vi "运维调试界面.vi"() -> ()   [LabVIEW 2016, in "质控单元V1.lvlib"]
uses:
  <vilib>/Utility/miscctls.llb/LVPointTypeDef.ctl
panel:
  in  "周期设置":bool
  in  "集成干预测试":bool
  in  "平行样测试":bool
  in  "水样测试":bool
  in  "数值":u8
  in  "向前寻道按钮":bool
  in  "向后寻道按钮":bool
  out "质控状态 4":T1
  out "质控状态 3":T1
  out "质控状态 2":T1
  out "质控状态":T1
  out "权限等级":string
  in  "布尔":bool
  out "模块版本号":string
  in  "停止":bool
  in  "参数设置":bool
  in  "连接设置":bool
  in  "调试界面":bool
  in  "加标回收":bool
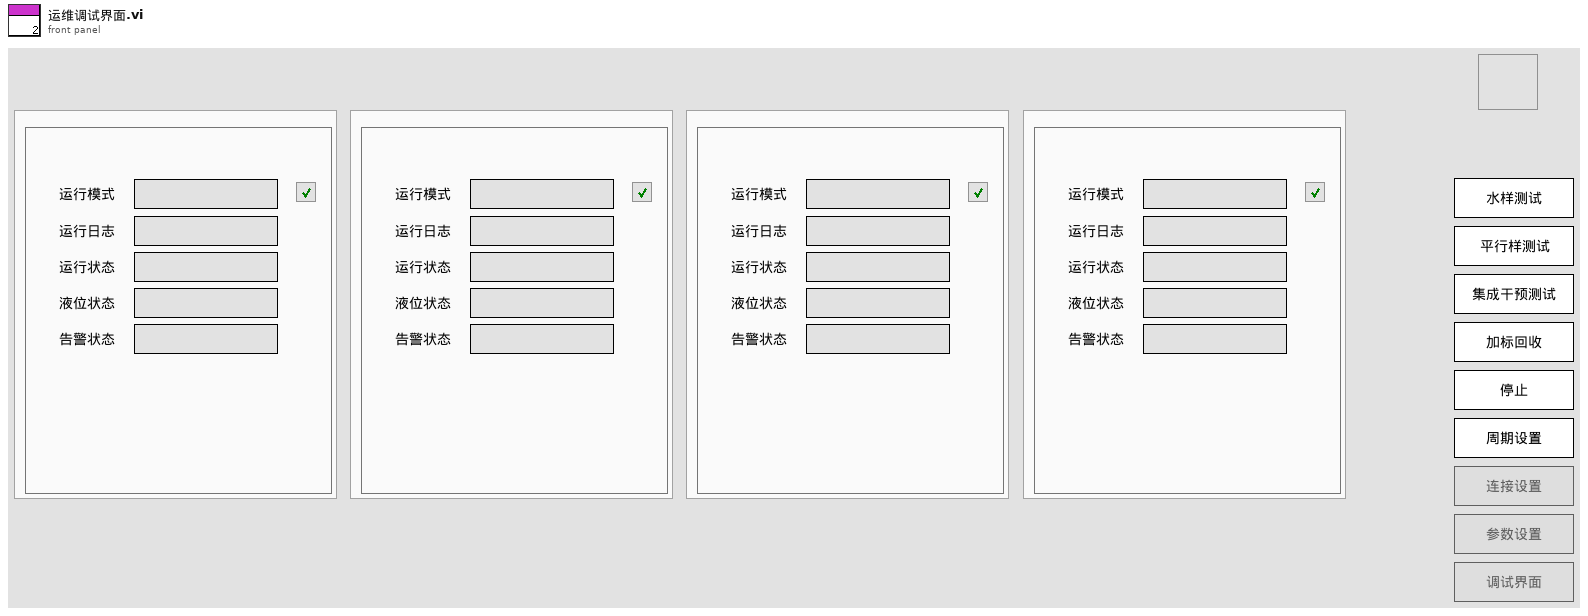
[diagram p1: front panel]
types:
  T1 = typedef "质控单元V1.lvlib/质控状态.ctl" = cluster{"模块名称":string, "通讯状态":bool, "运行模式":string, "运行日志":string, "运行状态":string, "液位状态":string, "告警状态":string}
  T2 = typedef "质控单元V1.lvlib/数据流类型.ctl" = cluster{"cmd":enum16{"start", "stop"}, "data":variant}
  T3 = typedef "LVPointTypeDef.ctl" = cluster{"Horizontal":i16, "Vertical":i16}
  T4 = typedef "质控单元V1.lvlib/质控仪器状态显示.ctl" = cluster{"运行模式":string, "运行状态":string, "液位状态":string, "告警状态":string, "加标体积":string}
  T5 = cluster{"氨氮":bool, "总磷":bool, "总氮":bool, "CODMn":bool, "CODCr":bool, "氨氮总磷":bool, "总磷总氮":bool}
  T6 = typedef "质控单元V1.lvlib/质控slave id.ctl" = enum16{"null", "氨氮", "总磷", "CODMn", "CODCr", "总氮"}
  T7 = typedef "质控单元V1.lvlib/测试流程.ctl" = enum16{"加标回收（启动采配水）", "加标回收（不启动采配水）", "水样测试（启动采配水）", "水样测试（不启动采配水）", "平行样测试（启动采配水）", "平行样测试（不启动采配水）", "集成干预测试"}
  T8 = cluster{"启用参数选择":cluster{"氨氮启用":bool, "总磷启用":bool, "总氮启用":bool, "CODMn启用":bool, "CODCr启用":bool}, "流程":T7}
  T9 = cluster{"氨氮启用":bool, "总磷启用":bool, "总氮启用":bool, "CODMn启用":bool, "CODCr启用":bool}
  T10 = enum8{"Enabled", "Disabled", "Disabled and Grayed Out"}
  T11 = cluster{"Major":u16, "Minor":u16, "Fix":u16, "Build":u16}
  T12 = cluster{"氨氮":bool, "总磷":bool, "总氮":bool, "CODMn":bool, "CODCr":bool}
  T13 = cluster{"氨氮":bool, "总磷":bool, "总氮":bool, "CODMn":bool, "CODCr":bool, bool}
  T14 = typedef "ZKTimingControl.lvlib/TimingControl.lvclass/国标控制命令.ctl" = enum16{"加标回收（启动采配水）", "加标回收（不启动采配水）", "水样测试（启动采配水）", "水样测试（不启动采配水）", "平行样测试（启动采配水）", "平行样测试（不启动采配水）", "集成干预测试"}
  T15 = typedef "ZKTimingControl.lvlib/TimingControl.lvclass/测量参数.ctl" = cluster{"氨氮":bool, "总磷":bool, "总氮":bool, "CODMn":bool, "CODCr":bool, "氟化物":bool}
  T16 = enum32{"Bad", "Idle", "Run top level", "Running"}
  T17 = cluster{"启动参数":cluster{"氨氮启用":bool, "总磷启用":bool, "总氮启用":bool, "CODMn启用":bool, "CODCr启用":bool}, "流程参数":T7}
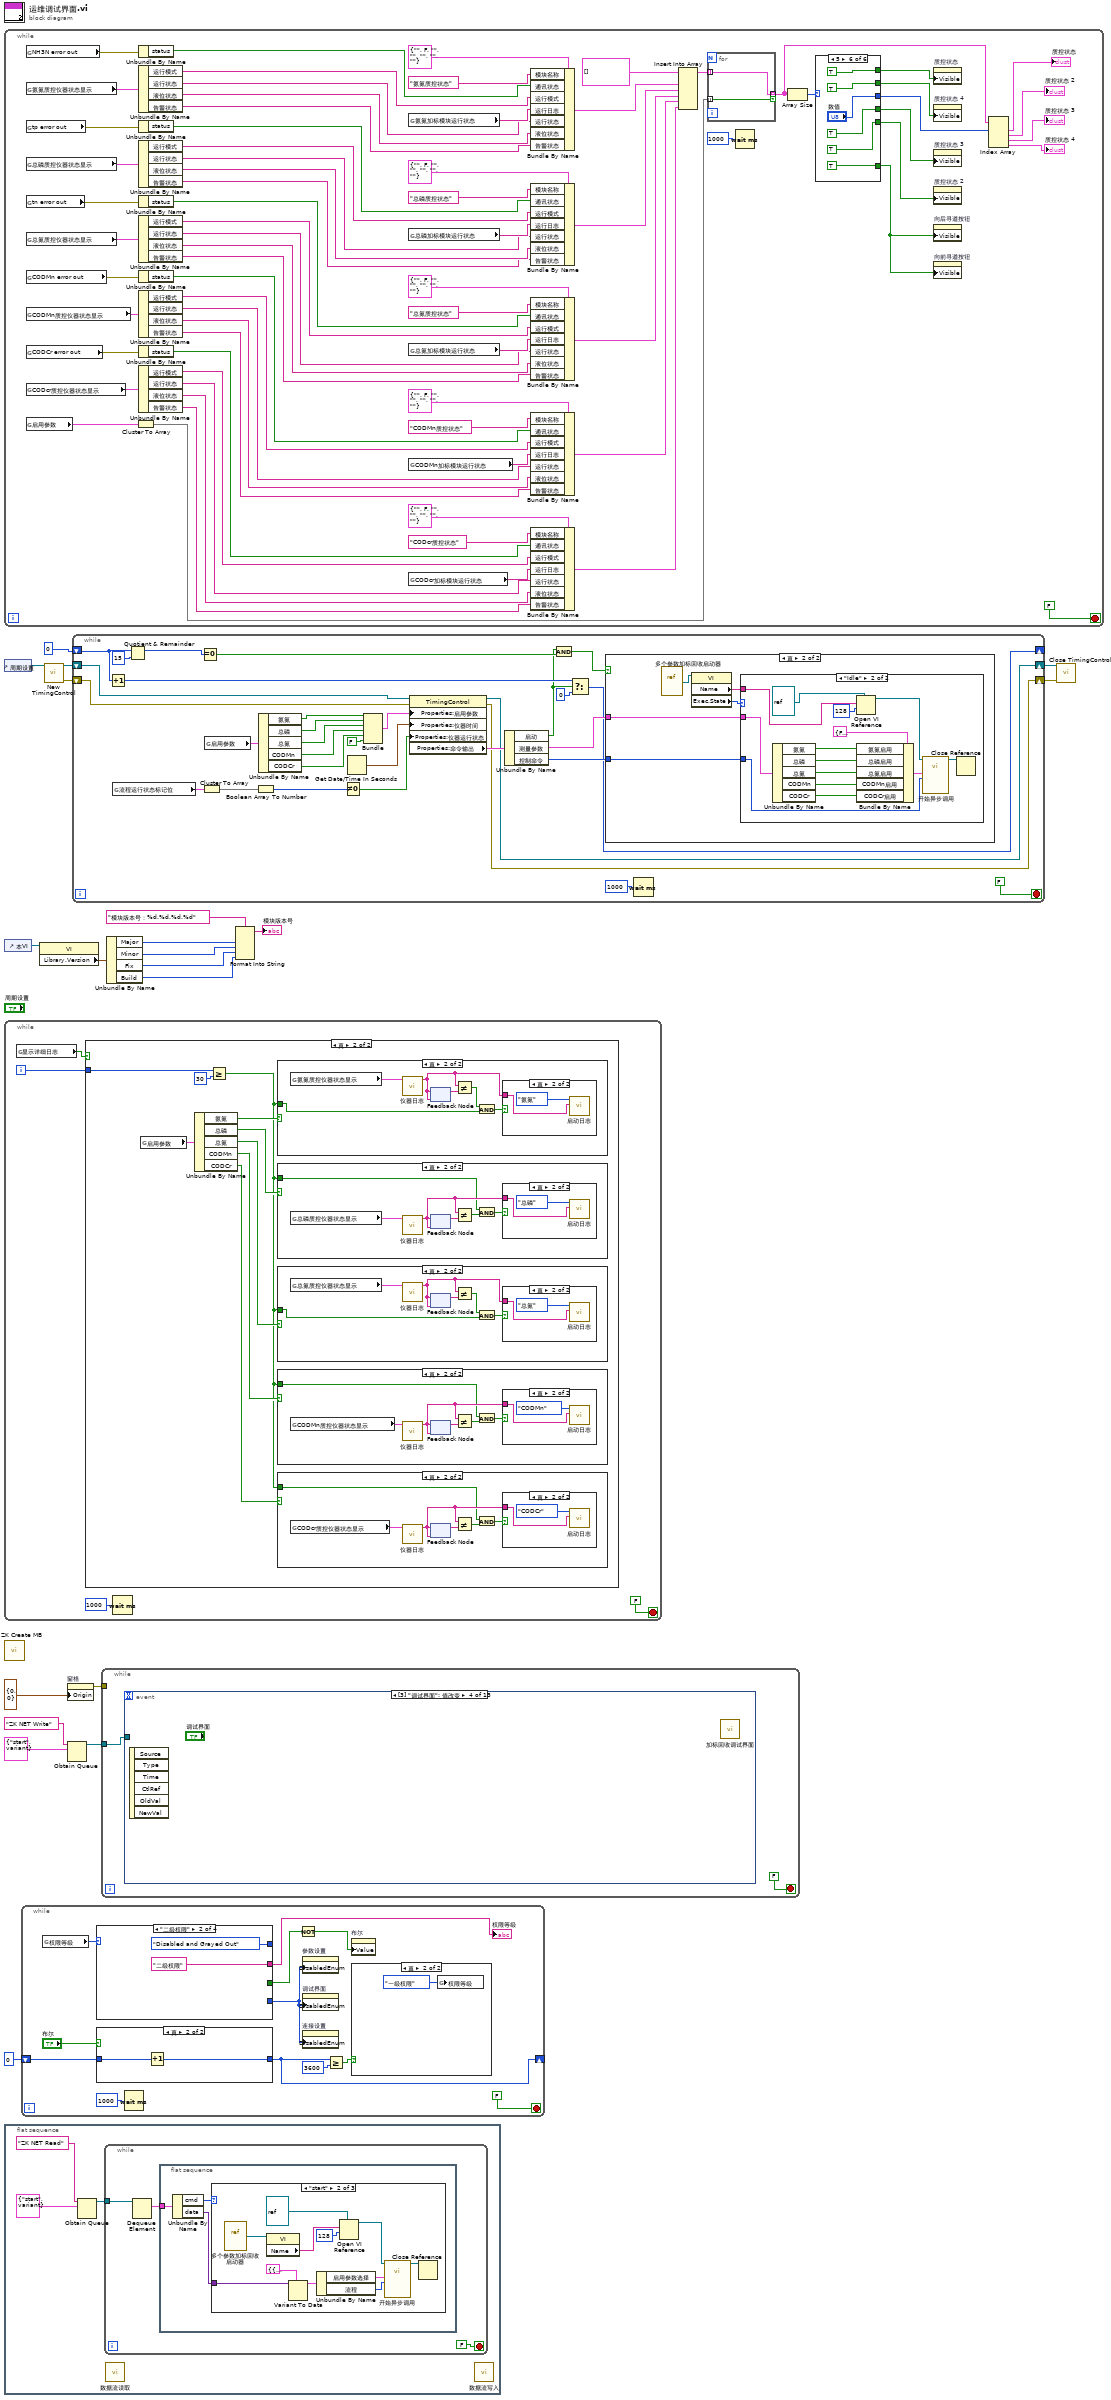
[diagram p0: block diagram]
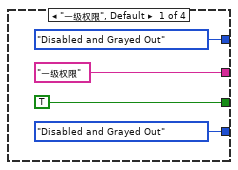
[diagram p13: hidden frame]
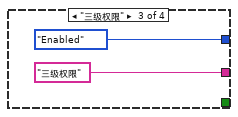
[diagram p14: hidden frame]
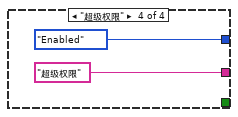
[diagram p15: hidden frame]
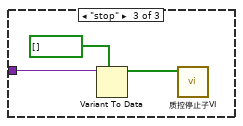
[diagram p19: hidden frame]
diagram:
  n1 = while {
    stop <- FALSE stop-if-true
    n2 = global read "ZK非断电保存全局变量.vi" "NH3N error out"() -> (w90:errorcluster)
    n3 = global read "ZK非断电保存全局变量.vi" "氨氮质控仪器状态显示"() -> (w89:T4)
    n4 = global read "ZK非断电保存全局变量.vi" "tp error out"() -> (w85:errorcluster)
    n5 = global read "ZK非断电保存全局变量.vi" "总磷质控仪器状态显示"() -> (w88:T4)
    n6 = global read "ZK非断电保存全局变量.vi" "tn error out"() -> (w84:errorcluster)
    n7 = global read "ZK非断电保存全局变量.vi" "总氮质控仪器状态显示"() -> (w87:T4)
    n8 = global read "ZK非断电保存全局变量.vi" "CODMn error out"() -> (w91:errorcluster)
    n9 = global read "ZK非断电保存全局变量.vi" "CODMn质控仪器状态显示"() -> (w86:T4)
    n10 = global read "ZK非断电保存全局变量.vi" "CODCr error out"() -> (w37:errorcluster)
    n11 = global read "ZK非断电保存全局变量.vi" "CODcr质控仪器状态显示"() -> (w38:T4)
    n12 = global read "ZK断电保存全局变量.vi" "启用参数"() -> (w34:T5)
    n13 = Cluster To Array(cluster=w34) -> (array=w33:bool[])
    n14 = Unbundle By Name(w90) -> ("status"=w82:bool)
    n15 = Unbundle By Name(w89) -> ("运行模式"=w80:string, "运行状态"=w78:string, "液位状态"=w77:string, "告警状态"=w76:string)
    n16 = Unbundle By Name(w85) -> ("status"=w68:bool)
    n17 = Unbundle By Name(w88) -> ("运行模式"=w73:string, "运行状态"=w72:string, "液位状态"=w71:string, "告警状态"=w70:string)
    n18 = Unbundle By Name(w84) -> ("status"=w55:bool)
    n19 = Unbundle By Name(w87) -> ("运行模式"=w57:string, "运行状态"=w54:string, "液位状态"=w53:string, "告警状态"=w52:string)
    n20 = Unbundle By Name(w91) -> ("status"=w65:bool)
    n21 = Unbundle By Name(w86) -> ("运行模式"=w63:string, "运行状态"=w62:string, "液位状态"=w61:string, "告警状态"=w60:string)
    n22 = Unbundle By Name(w37) -> ("status"=w41:bool)
    n23 = Unbundle By Name(w38) -> ("运行模式"=w43:string, "运行状态"=w44:string, "液位状态"=w45:string, "告警状态"=w46:string)
    n24 = global read "ZK非断电保存全局变量.vi" "氨氮加标模块运行状态"() -> (w79:string)
    n25 = global read "ZK非断电保存全局变量.vi" "总磷加标模块运行状态"() -> (w74:string)
    n26 = global read "ZK非断电保存全局变量.vi" "总氮加标模块运行状态"() -> (w56:string)
    n27 = global read "ZK非断电保存全局变量.vi" "CODMn加标模块运行状态"() -> (w64:string)
    n28 = global read "ZK非断电保存全局变量.vi" "CODcr加标模块运行状态"() -> (w42:string)
    n29 = Bundle By Name(cluster=T1 {"模块名称"="", "通讯状态"=FALSE, "运行模式"="", "运行日志"="", "运行状态"="", "液位状态"="", "告警状态"=""} ("质控状态"), "模块名称"="氨氮质控状态", "通讯状态"=w82, "运行模式"=w80, "运行日志"=w79, "运行状态"=w78, "液位状态"=w77, "告警状态"=w76) -> (w51:T1)
    n30 = Bundle By Name(cluster=T1 {"模块名称"="", "通讯状态"=FALSE, "运行模式"="", "运行日志"="", "运行状态"="", "液位状态"="", "告警状态"=""} ("质控状态"), "模块名称"="总磷质控状态", "通讯状态"=w68, "运行模式"=w73, "运行日志"=w74, "运行状态"=w72, "液位状态"=w71, "告警状态"=w70) -> (w49:T1)
    n31 = Bundle By Name(cluster=T1 {"模块名称"="", "通讯状态"=FALSE, "运行模式"="", "运行日志"="", "运行状态"="", "液位状态"="", "告警状态"=""} ("质控状态"), "模块名称"="总氮质控状态", "通讯状态"=w55, "运行模式"=w57, "运行日志"=w56, "运行状态"=w54, "液位状态"=w53, "告警状态"=w52) -> (w48:T1)
    n32 = Bundle By Name(cluster=T1 {"模块名称"="", "通讯状态"=FALSE, "运行模式"="", "运行日志"="", "运行状态"="", "液位状态"="", "告警状态"=""} ("质控状态"), "模块名称"="CODMn质控状态", "通讯状态"=w65, "运行模式"=w63, "运行日志"=w64, "运行状态"=w62, "液位状态"=w61, "告警状态"=w60) -> (w47:T1)
    n33 = Bundle By Name(cluster=T1 {"模块名称"="", "通讯状态"=FALSE, "运行模式"="", "运行日志"="", "运行状态"="", "液位状态"="", "告警状态"=""} ("质控状态"), "模块名称"="CODcr质控状态", "通讯状态"=w41, "运行模式"=w43, "运行日志"=w42, "运行状态"=w44, "液位状态"=w45, "告警状态"=w46) -> (w36:T1)
    n34 = Insert Into Array(array=T1[] [] ("数组"), new element #1=w51, new element #2=w49, new element #3=w48, new element #4=w47, new element #5=w36) -> (w35:T1[])  [unwired: 1 in]
    n35 = for {
      tunnel: w35 -> [w115] mode=indexing
      tunnel: w33 -> [w114] mode=indexing
      tunnel: [w115] -> w28 mode=indexing if=w114
    }
    n36 = Wait (ms)(milliseconds to wait=u32 1000 ("等待时间（毫秒）")) -> ()  [unwired: 1 out]
    n37 = Array Size(array=w28) -> (size(s)=w27:i32)
    n38 = case shown="5" w27 {
      tunnel: [FALSE TRUE TRUE TRUE TRUE TRUE] -> w26
      tunnel: [FALSE _ TRUE TRUE TRUE TRUE] -> w25
      tunnel: [FALSE _ _ TRUE TRUE TRUE] -> w24
      tunnel: [FALSE _ _ _ TRUE TRUE] -> w23
      tunnel: [_ _ _ _ _ TRUE] -> w22
      tunnel: [_ _ _ _ _ "数值"] -> w21
      frame 0, Default {
      }
      frame 1 {
      }
      frame 2 {
      }
      frame 3 {
      }
      frame 4 {
      }
      frame 5 {
      }
    }
    n39 = property on="质控状态" class="Clust (严格)"("Visible"=w26) -> ()  [unwired: 2 in, 2 out]
    n40 = property on="质控状态 4" class="Clust (严格)"("Visible"=w23) -> ()  [unwired: 2 in, 2 out]
    n41 = property on="质控状态 3" class="Clust (严格)"("Visible"=w24) -> ()  [unwired: 2 in, 2 out]
    n42 = property on="质控状态 2" class="Clust (严格)"("Visible"=w25) -> ()  [unwired: 2 in, 2 out]
    n43 = property on="向后寻道按钮" class="Bool"("Visible"=w22) -> ()  [unwired: 2 in, 2 out]
    n44 = property on="向前寻道按钮" class="Bool"("Visible"=w22) -> ()  [unwired: 2 in, 2 out]
    n45 = Index Array(array=w28, index #1=w21) -> (element #1=→"质控状态":T1, element #2=→"质控状态 2":T1, element #3=→"质控状态 3":T1, element #4=→"质控状态 4":T1)  [unwired: 3 in]
  }
  n46 = control-ref of="周期设置"() -> (w5:refnum<vi>)
  n47 = control-ref of="本VI"() -> (w18:refnum<vi>)
  n48 = while {
    i -> [w117]
    stop <- FALSE stop-if-true
    n49 = global read "ZK断电保存全局变量.vi" "显示详细日志"() -> (w116:bool)
    n50 = case shown="真" w116 {
      tunnel: w117 -> [_ w122]
      frame False {
      }
      frame True {
        n51 = global read "ZK断电保存全局变量.vi" "启用参数"() -> (w128:T5)
        n52 = Unbundle By Name(w128) -> ("氨氮"=w127:bool, "总磷"=w126:bool, "总氮"=w125:bool, "CODMn"=w124:bool, "CODCr"=w123:bool)
        n53 = Greater Or Equal?(x=w122, y=30) -> (x >= y?=w120:bool)
        n54 = case shown="真" w127 {
          tunnel: w120 -> [_ w161]
          frame False {
          }
          frame True {
            n55 = global read "ZK非断电保存全局变量.vi" "氨氮质控仪器状态显示"() -> (w166:T4)
            n56 = call "仪器日志.vi"("质控仪器状态显示"=w166) -> ("仪器日志"=w164:string)  [unwired: 10 in]
            n57 = feedback-in #1(w164) -> ()
            n58 = feedback #1(w164) -> (w165:string)
            n59 = Not Equal?(x=w164, y=w165) -> (x != y?=w163:bool)
            n60 = And(x=w163, y=w161) -> (x .and. y?=w162:bool)
            n61 = case shown="真" w162 {
              tunnel: w164 -> [_ w167]
              frame False {
              }
              frame True {
                n62 = call "启动日志.vi"("日志信息"=w167, "Slave ID"=质控slave_id."氨氮") -> ()  [unwired: 9 in, 1 out]
              }
            }
          }
        }
        n63 = case shown="真" w126 {
          tunnel: w120 -> [_ w153]
          frame False {
          }
          frame True {
            n64 = global read "ZK非断电保存全局变量.vi" "总磷质控仪器状态显示"() -> (w155:T4)
            n65 = call "仪器日志.vi"("质控仪器状态显示"=w155) -> ("仪器日志"=w157:string)  [unwired: 10 in]
            n66 = feedback #2(w157) -> (w158:string)
            n67 = feedback-in #2(w157) -> ()
            n68 = Not Equal?(x=w157, y=w158) -> (x != y?=w156:bool)
            n69 = And(x=w153, y=w156) -> (x .and. y?=w154:bool)
            n70 = case shown="真" w154 {
              tunnel: w157 -> [_ w159]
              frame False {
              }
              frame True {
                n71 = call "启动日志.vi"("日志信息"=w159, "Slave ID"=质控slave_id."总磷") -> ()  [unwired: 9 in, 1 out]
              }
            }
          }
        }
        n72 = case shown="真" w125 {
          tunnel: w120 -> [_ w145]
          frame False {
          }
          frame True {
            n73 = global read "ZK非断电保存全局变量.vi" "总氮质控仪器状态显示"() -> (w147:T4)
            n74 = call "仪器日志.vi"("质控仪器状态显示"=w147) -> ("仪器日志"=w149:string)  [unwired: 10 in]
            n75 = feedback #3(w149) -> (w150:string)
            n76 = feedback-in #3(w149) -> ()
            n77 = Not Equal?(x=w149, y=w150) -> (x != y?=w148:bool)
            n78 = And(x=w148, y=w145) -> (x .and. y?=w146:bool)
            n79 = case shown="真" w146 {
              tunnel: w149 -> [_ w151]
              frame False {
              }
              frame True {
                n80 = call "启动日志.vi"("日志信息"=w151, "Slave ID"=质控slave_id."总氮") -> ()  [unwired: 9 in, 1 out]
              }
            }
          }
        }
        n81 = case shown="真" w124 {
          tunnel: w120 -> [_ w137]
          frame False {
          }
          frame True {
            n82 = global read "ZK非断电保存全局变量.vi" "CODMn质控仪器状态显示"() -> (w139:T4)
            n83 = call "仪器日志.vi"("质控仪器状态显示"=w139) -> ("仪器日志"=w141:string)  [unwired: 10 in]
            n84 = feedback #4(w141) -> (w142:string)
            n85 = feedback-in #4(w141) -> ()
            n86 = Not Equal?(x=w141, y=w142) -> (x != y?=w140:bool)
            n87 = And(x=w137, y=w140) -> (x .and. y?=w138:bool)
            n88 = case shown="真" w138 {
              tunnel: w141 -> [_ w143]
              frame False {
              }
              frame True {
                n89 = call "启动日志.vi"("日志信息"=w143, "Slave ID"=质控slave_id."CODMn") -> ()  [unwired: 9 in, 1 out]
              }
            }
          }
        }
        n90 = case shown="真" w123 {
          tunnel: w120 -> [_ w129]
          frame False {
          }
          frame True {
            n91 = global read "ZK非断电保存全局变量.vi" "CODcr质控仪器状态显示"() -> (w131:T4)
            n92 = call "仪器日志.vi"("质控仪器状态显示"=w131) -> ("仪器日志"=w133:string)  [unwired: 10 in]
            n93 = feedback #5(w133) -> (w134:string)
            n94 = feedback-in #5(w133) -> ()
            n95 = Not Equal?(x=w133, y=w134) -> (x != y?=w132:bool)
            n96 = And(x=w129, y=w132) -> (x .and. y?=w130:bool)
            n97 = case shown="真" w130 {
              tunnel: w133 -> [_ w135]
              frame False {
              }
              frame True {
                n98 = call "启动日志.vi"("日志信息"=w135, "Slave ID"=质控slave_id."CODCr") -> ()  [unwired: 9 in, 1 out]
              }
            }
          }
        }
      }
    }
    n99 = Wait (ms)(milliseconds to wait=u32 1000 ("等待时间（毫秒）")) -> ()  [unwired: 1 out]
  }
  n100 = call "ZK Create MB.vi"() -> ()  [unwired: 12 in]
  n101 = flat-sequence {
    frame #0 {
      n102 = Obtain Queue(name (unnamed)="ZK NET Read" ("名称（未命名）"), element data type=T2 {"cmd"=enum."start", "data"=variant} ("簇")) -> (queue out=w170:refnum<queue>)  [unwired: 3 in, 2 out]
      n103 = while {
        tunnel: w170 -> [w174]
        stop <- FALSE stop-if-true
        n104 = Dequeue Element(queue=w174) -> (element=w172:T2)  [unwired: 2 in, 3 out]
        n105 = flat-sequence {
          tunnel: w172 -> [w177]
          frame #0 {
            n106 = Unbundle By Name(w177) -> ("cmd"=w176:enum16{"start", "stop"}, "data"=w175:variant)
            n107 = case shown="\"start\"" w176 {
              tunnel: w175 -> [_ w180 w191]
              frame Default {
              }
              frame "start" {
                n108 = vi-ref "多个参数加标回收启动器.vi"() -> (w188:refnum<vi>)
                n109 = property class="VI"(reference=w188) -> ("Name"=w187:string)  [unwired: 1 in, 2 out]
                n110 = Variant To Data(type=T8 {"启用参数选择"={"氨氮启用"=FALSE, "总磷启用"=FALSE, "总氮启用"=FALSE, "CODMn启用"=FALSE, "CODCr启用"=FALSE}, "流程"=enum."加标回收（启动采配水）"} ("data"), Variant=w180) -> (data=w182:T8)  [unwired: 1 in, 1 out]
                n111 = Unbundle By Name(w182) -> ("启用参数选择"=w181:T9, "流程"=w178:T7)
                n112 = Open VI Reference(type specifier VI Refnum (for type only)=refnum<vi> refnum, vi path=w187, options=128 ("选项")) -> (vi reference=w185:refnum<vi>)  [unwired: 3 in, 1 out]
                n113 = call-by-ref "开始异步调用"(reference=w185, "流程"=w178, "启用参数选择"=w181) -> (reference out=w184:refnum<vi>)  [unwired: 11 in, 1 out]
                n114 = Close Reference(reference=w184) -> ()  [unwired: 1 in, 1 out]
              }
              frame "stop" {
                n115 = Variant To Data(type=bool[] [] ("数组"), Variant=w191) -> (data=w189:bool[])  [unwired: 1 in, 1 out]
                n116 = call "质控停止子VI.vi"("数组"=w189) -> ()  [unwired: 11 in]
              }
            }
          }
        }
      }
      n117 = call "数据流读取.vi"() -> ()  [unwired: 12 in]
      n118 = call "数据流写入.vi"() -> ()  [unwired: 12 in]
    }
  }
  n119 = while {
    shift-right: [w202] -> _
    shift-left: 0 -> [w203]
    stop <- FALSE stop-if-true
    n120 = global read "ZK非断电保存全局变量.vi" "权限等级"() -> (w197:enum16{"一级权限", "二级权限", "三级权限", "超级权限"})
    n121 = case shown="\"二级权限\"" w197 {
      tunnel: [T10."Disabled and Grayed Out" ("禁用") _ _ _] -> w192
      tunnel: ["一级权限" "二级权限" "三级权限" "超级权限"] -> w195
      tunnel: [TRUE ("布尔") _ _ _] -> w194
      tunnel: [T10."Disabled and Grayed Out" ("禁用") T10."Disabled and Grayed Out" ("禁用") T10."Enabled" ("禁用") T10."Enabled" ("禁用")] -> _
      frame "一级权限", Default {
      }
      frame "二级权限" {
      }
      frame "三级权限" {
      }
      frame "超级权限" {
      }
    }
    "权限等级" <- w195
    n122 = case shown="真" "布尔" {
      tunnel: w203 -> [_ w216]
      tunnel: [_ w215] -> w202
      frame False {
      }
      frame True {
        n123 = Increment(x=w216) -> (x+1=w215:i32)
      }
    }
    n124 = Wait (ms)(milliseconds to wait=u32 1000 ("等待时间（毫秒）")) -> ()  [unwired: 1 out]
    n125 = Not(x=w194) -> (.not. x?=w193:bool)
    n126 = property on="参数设置" class="Bool"("DisabledEnum"=w192) -> ()  [unwired: 2 in, 2 out]
    n127 = property on="调试界面" class="Bool"("DisabledEnum"=w192) -> ()  [unwired: 2 in, 2 out]
    n128 = property on="连接设置" class="Bool"("DisabledEnum"=w192) -> ()  [unwired: 2 in, 2 out]
    n129 = Greater Or Equal?(x=w202, y=3600) -> (x >= y?=w200:bool)
    n130 = property on="布尔" class="Bool (严格)"("Value"=w193) -> ()  [unwired: 2 in, 2 out]
    n131 = case shown="真" w200 {
      frame False {
      }
      frame True {
        n132 = global write "ZK非断电保存全局变量.vi" "权限等级"(enum16{"一级权限", "二级权限", "三级权限", "超级权限"}."一级权限" ("权限等级")) -> ()
      }
    }
  }
  n133 = property class="VI"(reference=w18) -> ("Library.Version"=w17:T11)  [unwired: 1 in, 2 out]
  n134 = call "New TimingControl.vi"("Reference"=w5) -> ("error out"=w3:errorcluster, "TimingControl out"=w4:refnum<class "TimingControl.lvclass">)  [unwired: 9 in]
  n135 = property on="窗格" class="Pane"("Origin"=T3 {"Horizontal"=0, "Vertical"=0} ("原点")) -> (error out=w19:errorcluster)  [unwired: 2 in, 1 out]
  n136 = Obtain Queue(name (unnamed)="ZK NET Write" ("名称（未命名）"), element data type=T2 {"cmd"=enum."start", "data"=variant} ("簇")) -> (queue out=w9:refnum<queue>)  [unwired: 3 in, 2 out]
  n137 = while {
    shift-right: [w232] -> _
    shift-left: 0 -> [w231]
    shift-right: [w218] -> w2
    shift-left: w4 -> [w225]
    shift-right: [w217] -> w1
    shift-left: w3 -> [w224]
    stop <- FALSE stop-if-true
    n138 = Increment(x=w231) -> (x+1=w234:i32)
    n139 = global read "ZK非断电保存全局变量.vi" "流程运行状态标记位"() -> (w243:T12)
    n140 = Quotient & Remainder(x=w231, y=15) -> (x-y*floor(x/y)=w229:i32)  [unwired: 1 out]
    n141 = Equal To 0?(x=w229) -> (x = 0?=w228:bool)
    n142 = Cluster To Array(cluster=w243) -> (array=w242:bool[])
    n143 = global read "ZK断电保存全局变量.vi" "启用参数"() -> (w240:T5)
    n144 = Boolean Array To Number(Boolean array=w242) -> (number=w241:u32)
    n145 = Unbundle By Name(w240) -> ("氨氮"=w239:bool, "总磷"=w238:bool, "总氮"=w237:bool, "CODMn"=w236:bool, "CODCr"=w235:bool)
    n146 = Not Equal To 0?(x=w241) -> (x != 0?=w219:bool)
    n147 = Get Date/Time In Seconds() -> (seconds since 1Jan1904=w220:timestamp)
    n148 = Bundle("氨氮"=w239, "总磷"=w238, "总氮"=w237, "CODMn"=w236, "CODCr"=w235, FALSE) -> (w222:T13)  [unwired: 1 in]
    n149 = property class="TimingControl"(reference=w225, error in=w224, "Properties:启用参数"=w222, "Properties:仪器时间"=w220, "Properties:仪器运行状态"=w219) -> (reference out=w218:refnum<class "TimingControl.lvclass">, error out=w217:errorcluster, "Properties:命令输出"=w223:cluster{"启动":bool, "控制命令":T14, "测量参数":T15})
    n150 = Unbundle By Name(w223) -> ("启动"=w227:bool, "测量参数"=w245:T15, "控制命令"=w244:T14)
    n151 = And(x=w227, y=w228) -> (x .and. y?=w226:bool)
    n152 = Select(t=w234, s=w227, f=0) -> (s? t:f=w232:i32)
    n153 = case shown="真" w226 {
      tunnel: w245 -> [_ w250]
      tunnel: w244 -> [_ w249]
      frame False {
      }
      frame True {
        n154 = vi-ref "多个参数加标回收启动器.vi"() -> (w251:refnum<vi>)
        n155 = property class="VI"(reference=w251) -> ("Name"=w252:string, "Exec.State"=w248:T16)  [unwired: 1 in, 2 out]
        n156 = case shown="\"Idle\"" w248 {
          tunnel: w252 -> [_ w263]
          tunnel: w250 -> [_ w258]
          tunnel: w249 -> [_ w262]
          frame "Bad", Default {
          }
          frame "Idle" {
            n157 = Unbundle By Name(w258) -> ("氨氮"=w257:bool, "总磷"=w256:bool, "总氮"=w255:bool, "CODMn"=w254:bool, "CODCr"=w253:bool)
            n158 = Bundle By Name(cluster=T9 {"氨氮启用"=FALSE, "总磷启用"=FALSE, "总氮启用"=FALSE, "CODMn启用"=FALSE, "CODCr启用"=FALSE} ("启用参数选择"), "氨氮启用"=w257, "总磷启用"=w256, "总氮启用"=w255, "CODMn启用"=w254, "CODCr启用"=w253) -> (w259:T9)
            n159 = Open VI Reference(type specifier VI Refnum (for type only)=refnum<vi> refnum, vi path=w263, options=128 ("选项")) -> (vi reference=w265:refnum<vi>)  [unwired: 3 in, 1 out]
            n160 = call-by-ref "开始异步调用"(reference=w265, "流程"=w262, "启用参数选择"=w259) -> (reference out=w266:refnum<vi>)  [unwired: 11 in, 1 out]
            n161 = Close Reference(reference=w266) -> ()  [unwired: 1 in, 1 out]
          }
        }
      }
    }
    n162 = Wait (ms)(milliseconds to wait=u32 1000 ("等待时间（毫秒）")) -> ()  [unwired: 1 out]
  }
  n163 = while {
    tunnel: w19 -> [_]
    tunnel: w9 -> [w267]
    stop <- FALSE stop-if-true
    n164 = event shown="[3] \"调试界面\": 值改变" {
      selector: _ -> [_ _ _ _ _ _ _ _ _ _ _ _ _]
      dyn-events: _ -> [_ _ _ _ _ _ _ _ _ _ _ _ _]
      timeout: _ -> [_ _ _ _ _ _ _ _ _ _ _ _ _]
      tunnel: w267 -> [_ _ _ _ _ _ _ w280 w298 w316 w334 w354 _]
      event Timeout {
        n165 = event-data() -> ()  [unwired: 1 in, 3 out]
      }
      event "布尔": Value Change {
        n166 = event-data() -> ("NewVal"=w269:bool)  [unwired: 1 in, 3 out]
        n167 = case shown="真" w269 {
          frame False {
            n168 = global write "ZK非断电保存全局变量.vi" "权限等级"(enum16{"一级权限", "二级权限", "三级权限", "超级权限"}."一级权限" ("权限等级")) -> ()
          }
          frame True {
            n169 = global read "ZK非断电保存全局变量.vi" "权限密码"() -> (w273:u32[])
            n170 = global read "ZK非断电保存全局变量.vi" "权限等级"() -> (w271:enum16{"一级权限", "二级权限", "三级权限", "超级权限"})
            n171 = call "密码权限设置.vi"("权限输入"=w271, "权限密码"=w273) -> ("权限输出"=w272:enum16{"一级权限", "二级权限", "三级权限", "超级权限"})  [unwired: 9 in]
            n172 = global write "ZK非断电保存全局变量.vi" "权限等级"(w272) -> ()
          }
        }
      }
      event "权限等级": Mouse Down {
        n173 = event-data() -> ()  [unwired: 1 in, 8 out]
        n174 = global read "ZK非断电保存全局变量.vi" "权限密码"() -> (w276:u32[])
        n175 = global read "ZK非断电保存全局变量.vi" "权限等级"() -> (w274:enum16{"一级权限", "二级权限", "三级权限", "超级权限"})
        n176 = call "密码权限设置.vi"("权限输入"=w274, "权限密码"=w276) -> ("权限输出"=w275:enum16{"一级权限", "二级权限", "三级权限", "超级权限"})  [unwired: 9 in]
        n177 = global write "ZK非断电保存全局变量.vi" "权限等级"(w275) -> ()
      }
      event "调试界面": Value Change {
        n178 = event-data() -> ()  [unwired: 1 in, 6 out]
        n179 = call "加标回收调试界面.vi"() -> ()  [unwired: 12 in]
      }
      event "向后寻道按钮": Value Change {
        n180 = event-data() -> ()  [unwired: 1 in, 6 out]
        n181 = property on="数值" class="DigNum (严格)"("Value"=u8 1 ("数值")) -> ()  [unwired: 2 in, 2 out]
      }
      event "向前寻道按钮": Value Change {
        n182 = event-data() -> ()  [unwired: 1 in, 6 out]
        n183 = property on="数值" class="DigNum (严格)"("Value"=u8 0 ("数值")) -> ()  [unwired: 2 in, 2 out]
      }
      event "参数设置": Value Change {
        n184 = event-data() -> ()  [unwired: 1 in, 6 out]
        n185 = call "加标回收参数设置.vi"() -> ()  [unwired: 12 in]
      }
      event "加标回收": Value Change {
        n186 = event-data() -> ()  [unwired: 1 in, 6 out]
        n187 = call "加标回收启动对话框.vi"("测试模式"=enum16{"水样测试", "平行样测试", "加标回收", "集成干预测试"}."加标回收") -> ("流程参数"=w281:T7, "启动参数"=w282:T9, "check ？"=w283:bool)  [unwired: 8 in]
        n188 = case shown="真" w283 {
          tunnel: w282 -> [_ w290]
          tunnel: w281 -> [_ w289]
          tunnel: w280 -> [_ w291]
          frame False {
          }
          frame True {
            n189 = Bundle("启动参数"=w290, "流程参数"=w289) -> (w286:T17)  [unwired: 1 in]
            n190 = vi-ref "多个参数加标回收启动器.vi"() -> (w296:refnum<vi>)
            n191 = property class="VI"(reference=w296) -> ("Name"=w295:string)  [unwired: 1 in, 2 out]
            n192 = Bundle By Name(cluster=T2 {"cmd"=enum."start", "data"=variant} ("簇"), "cmd"=enum16{"start", "stop"}."start", "data"=w286) -> (w285:T2)
            n193 = Enqueue Element(queue=w291, element=w285) -> ()  [unwired: 2 in, 3 out]
            n194 = Open VI Reference(type specifier VI Refnum (for type only)=refnum<vi> refnum, vi path=w295, options=128 ("选项")) -> (vi reference=w293:refnum<vi>)  [unwired: 3 in, 1 out]
            n195 = call-by-ref "开始异步调用"(reference=w293, "流程"=w289, "启用参数选择"=w290) -> (reference out=w292:refnum<vi>)  [unwired: 11 in, 1 out]
            n196 = Close Reference(reference=w292) -> ()  [unwired: 1 in, 1 out]
          }
        }
      }
      event "水样测试": Value Change {
        n197 = event-data() -> ()  [unwired: 1 in, 6 out]
        n198 = call "加标回收启动对话框.vi"("测试模式"=enum16{"水样测试", "平行样测试", "加标回收", "集成干预测试"}."水样测试") -> ("流程参数"=w299:T7, "启动参数"=w300:T9, "check ？"=w301:bool)  [unwired: 8 in]
        n199 = case shown="真" w301 {
          tunnel: w300 -> [_ w308]
          tunnel: w299 -> [_ w307]
          tunnel: w298 -> [_ w309]
          frame False {
          }
          frame True {
            n200 = Bundle("启动参数"=w308, "流程参数"=w307) -> (w304:T17)  [unwired: 1 in]
            n201 = vi-ref "多个参数加标回收启动器.vi"() -> (w314:refnum<vi>)
            n202 = property class="VI"(reference=w314) -> ("Name"=w313:string)  [unwired: 1 in, 2 out]
            n203 = Bundle By Name(cluster=T2 {"cmd"=enum."start", "data"=variant} ("簇"), "cmd"=enum16{"start", "stop"}."start", "data"=w304) -> (w303:T2)
            n204 = Enqueue Element(queue=w309, element=w303) -> ()  [unwired: 2 in, 3 out]
            n205 = Open VI Reference(type specifier VI Refnum (for type only)=refnum<vi> refnum, vi path=w313, options=128 ("选项")) -> (vi reference=w311:refnum<vi>)  [unwired: 3 in, 1 out]
            n206 = call-by-ref "开始异步调用"(reference=w311, "流程"=w307, "启用参数选择"=w308) -> (reference out=w310:refnum<vi>)  [unwired: 11 in, 1 out]
            n207 = Close Reference(reference=w310) -> ()  [unwired: 1 in, 1 out]
          }
        }
      }
      event "平行样测试": Value Change {
        n208 = event-data() -> ()  [unwired: 1 in, 6 out]
        n209 = call "加标回收启动对话框.vi"("测试模式"=enum16{"水样测试", "平行样测试", "加标回收", "集成干预测试"}."平行样测试") -> ("流程参数"=w317:T7, "启动参数"=w318:T9, "check ？"=w319:bool)  [unwired: 8 in]
        n210 = case shown="真" w319 {
          tunnel: w318 -> [_ w326]
          tunnel: w317 -> [_ w325]
          tunnel: w316 -> [_ w327]
          frame False {
          }
          frame True {
            n211 = Bundle("启动参数"=w326, "流程参数"=w325) -> (w322:T17)  [unwired: 1 in]
            n212 = vi-ref "多个参数加标回收启动器.vi"() -> (w332:refnum<vi>)
            n213 = property class="VI"(reference=w332) -> ("Name"=w331:string)  [unwired: 1 in, 2 out]
            n214 = Bundle By Name(cluster=T2 {"cmd"=enum."start", "data"=variant} ("簇"), "cmd"=enum16{"start", "stop"}."start", "data"=w322) -> (w321:T2)
            n215 = Enqueue Element(queue=w327, element=w321) -> ()  [unwired: 2 in, 3 out]
            n216 = Open VI Reference(type specifier VI Refnum (for type only)=refnum<vi> refnum, vi path=w331, options=128 ("选项")) -> (vi reference=w329:refnum<vi>)  [unwired: 3 in, 1 out]
            n217 = call-by-ref "开始异步调用"(reference=w329, "流程"=w325, "启用参数选择"=w326) -> (reference out=w328:refnum<vi>)  [unwired: 11 in, 1 out]
            n218 = Close Reference(reference=w328) -> ()  [unwired: 1 in, 1 out]
          }
        }
      }
      event "集成干预测试": Value Change {
        n219 = event-data() -> ()  [unwired: 1 in, 6 out]
        n220 = call "加标回收启动对话框.vi"("测试模式"=enum16{"水样测试", "平行样测试", "加标回收", "集成干预测试"}."集成干预测试") -> ("流程参数"=w335:T7, "启动参数"=w336:T9, "check ？"=w337:bool)  [unwired: 8 in]
        n221 = case shown="真" w337 {
          tunnel: w336 -> [_ w344]
          tunnel: w335 -> [_ w343]
          tunnel: w334 -> [_ w345]
          frame False {
          }
          frame True {
            n222 = Bundle("启动参数"=w344, "流程参数"=w343) -> (w340:T17)  [unwired: 1 in]
            n223 = vi-ref "多个参数加标回收启动器.vi"() -> (w350:refnum<vi>)
            n224 = property class="VI"(reference=w350) -> ("Name"=w349:string)  [unwired: 1 in, 2 out]
            n225 = Bundle By Name(cluster=T2 {"cmd"=enum."start", "data"=variant} ("簇"), "cmd"=enum16{"start", "stop"}."start", "data"=w340) -> (w339:T2)
            n226 = Enqueue Element(queue=w345, element=w339) -> ()  [unwired: 2 in, 3 out]
            n227 = Open VI Reference(type specifier VI Refnum (for type only)=refnum<vi> refnum, vi path=w349, options=128 ("选项")) -> (vi reference=w347:refnum<vi>)  [unwired: 3 in, 1 out]
            n228 = call-by-ref "开始异步调用"(reference=w347, "流程"=w343, "启用参数选择"=w344) -> (reference out=w346:refnum<vi>)  [unwired: 11 in, 1 out]
            n229 = Close Reference(reference=w346) -> ()  [unwired: 1 in, 1 out]
          }
        }
      }
      event "停止": Value Change {
        n230 = event-data() -> ()  [unwired: 1 in, 6 out]
        n231 = Flush Queue(queue=w354) -> (queue out=w353:refnum<queue>)  [unwired: 1 in, 2 out]
        n232 = call "加标回收停止对话框.vi"() -> ("数组"=w352:bool[], "check？"=w351:bool)  [unwired: 10 in]
        n233 = case shown="真" w351 {
          tunnel: w353 -> [_ w359]
          tunnel: w352 -> [_ w355]
          frame False {
          }
          frame True {
            n234 = call "质控停止子VI.vi"("数组"=w355) -> ()  [unwired: 11 in]
            n235 = Bundle By Name(cluster=T2 {"cmd"=enum."start", "data"=variant} ("簇"), "cmd"=enum16{"start", "stop"}."stop", "data"=w355) -> (w356:T2)
            n236 = Enqueue Element(queue=w359, element=w356) -> ()  [unwired: 2 in, 3 out]
          }
        }
      }
      event "连接设置": Value Change {
        n237 = event-data() -> ()  [unwired: 1 in, 6 out]
        n238 = call "串口配置.vi"() -> ()  [unwired: 12 in]
      }
    }
  }
  n239 = Unbundle By Name(w17) -> ("Major"=w15:u16, "Minor"=w14:u16, "Fix"=w13:u16, "Build"=w12:u16)
  n240 = Format Into String(format string="模块版本号：%d.%d.%d.%d" ("格式字符串"), w15, w14, w13, w12) -> (resulting string=→"模块版本号":string)  [unwired: 2 in, 1 out]
  n241 = call "Close TimingControl.vi"("error in (no error)"=w1, "TimingControl in"=w2) -> ()  [unwired: 9 in, 1 out]
